vi "Choreo_ChoreoSwerve_AvailableTrajectories.vi"(8 "error in (no error)":errorcluster) -> (0 "error out":errorcluster, 3 "filenames":string[](array[string]))   [LabVIEW 2019, in "ChoreoLib.lvlib"]
doc: "Load a Choreo trajectory from a JSON formatted file. Note that for newer versions of Choreo, the file has a \".traj\" extension. Internally this is formatted as a JSON file.\n\nInputs: \n - filename - string - The name of the trajectory file. See notes below on file naming.\n\nOutputs:\n - Trajectory - cluster - Trajectory read from JSON file.\n - Error out - cluster - Error cluster\n - Full Filename - string - fully qualified file name.\n\nNotes on file naming:\n - The file name must include the extention. \".json\", or \".traj\" is not automatically appended to the name. \n - The file name can be a simple file or an absolute path. If a simple file name is used the default path on the RoboRIO is: \"home:\\lvuser\\natinst\\LabVIEW Data\". On a Windows PC the default path is the LabVIEW default directory. Normally this is: “%HOMEDRIVE%%HOMEPATH%\\Documents\\LabView Data\".\n - Filenames on the RoboRIO, which runs Linux, are case sensitive."
uses:
  ChoreoLib.lvlib
panel:
  out "Path Out":path
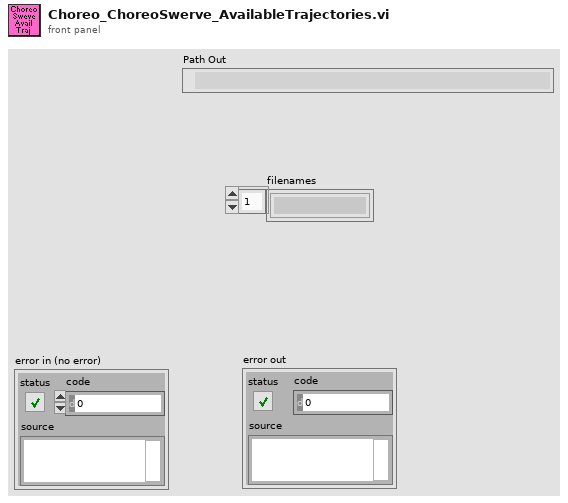
[diagram p1: front panel]
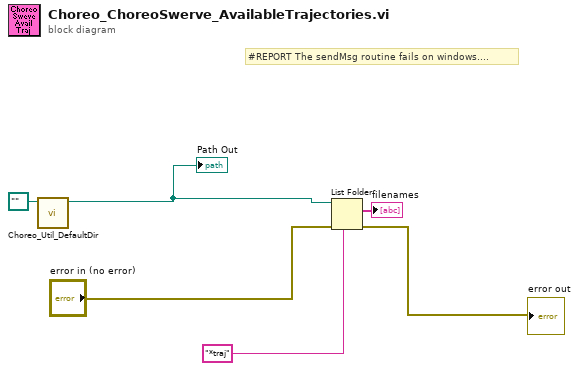
[diagram p0: block diagram]
diagram:
  # "#REPORT The sendMsg routine fails on windows...."
  n1 = call "Choreo_Util_DefaultDir.vi"("Path in"=path "") -> ("Path Out"=w5:path)  [unwired: 10 in]
  "Path Out" <- w5
  n2 = List Folder(path=w5, pattern="*traj", error in="error in (no error)") -> (filenames=→"filenames":string[], error out=→"error out":errorcluster)  [unwired: 1 in, 2 out]
